vi "Wärmepumpe.VorlauftemperaturSolekreislauf.vi"(0 "Wärmepumpe in":refnum<data-value>, 4 "Rücklauftemperatur Solekreislauf[°C]":dbl, 5 "Error in":errorcluster) -> (14 "Wärmepumpe out":refnum<data-value>, 19 "Error out":errorcluster)   [LabVIEW 2016, in "Wärmepumpe.lvclass"]
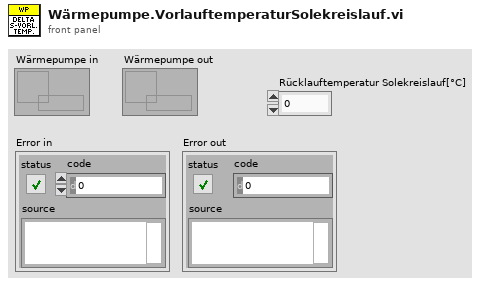
[diagram p1: front panel]
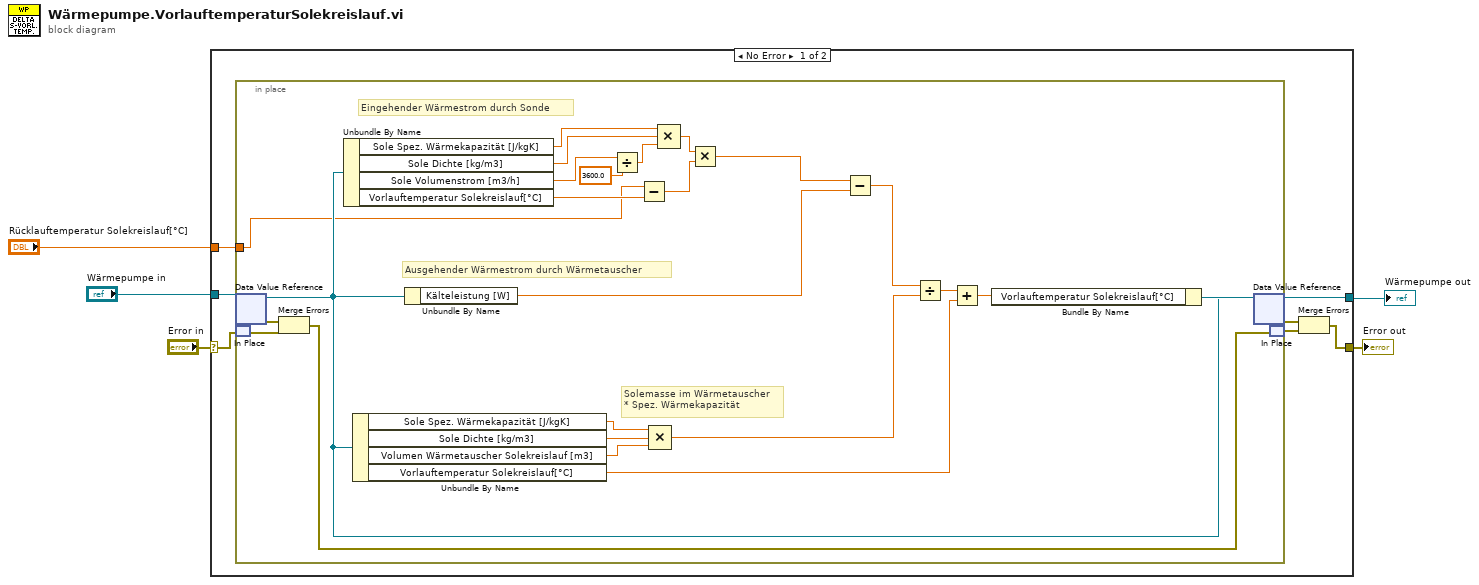
[diagram p0: block diagram]
diagram:
  n1 = case shown="No Error" "Error in" {
    selector: "Error in" -> [w10 w38]
    tunnel: [w9 w37] -> w4
    tunnel: [w8 w38] -> w3
    tunnel: "Wärmepumpe in" -> [w7 w37]
    tunnel: "Rücklauftemperatur Solekreislauf[°C]" -> [w6 _]
    frame No Error {
      n2 = in-place {
        in-place-border: w6 -> [w21]
        # "Solemasse im Wärmetauscher\n* Spez. Wärmekapazität"
        # "Eingehender Wärmestrom durch Sonde"
        # "Ausgehender Wärmestrom durch Wärmetauscher"
        n3 = in-place-dvr #1(w7) -> (w23:refnum<class "Wärmepumpe.lvclass">, w36:errorcluster)
        n4 = in-place-match #2(w10) -> (w35:errorcluster)
        n5 = Merge Errors(w36, w35) -> (w34:errorcluster)
        n6 = Unbundle By Name(w23) -> ("Sole Spez. Wärmekapazität [J/kgK]"=w17:dbl, "Sole Dichte [kg/m3]"=w16:dbl, "Sole Volumenstrom [m3/h]"=w15:dbl, "Vorlauftemperatur Solekreislauf[°C]"=w22:dbl)
        n7 = Unbundle By Name(w23) -> ("Sole Spez. Wärmekapazität [J/kgK]"=w19:dbl, "Sole Dichte [kg/m3]"=w20:dbl, "Volumen Wärmetauscher Solekreislauf [m3]"=w25:dbl, "Vorlauftemperatur Solekreislauf[°C]"=w29:dbl)
        n8 = Unbundle By Name(w23) -> ("Kälteleistung [W]"=w13:dbl)
        n9 = Divide(x=w15, y=3600.0) -> (x/y=w14:dbl)
        n10 = Subtract(x=w21, y=w22) -> (x-y=w26:dbl)
        n11 = Compound Arithmetic op=MULTIPLY(w19, w20, w25) -> (w28:dbl)
        n12 = Compound Arithmetic op=MULTIPLY(w17, w16, w14) -> (w27:dbl)
        n13 = Multiply(x=w27, y=w26) -> (x*y=w24:dbl)
        n14 = Subtract(x=w24, y=w13) -> (x-y=w33:dbl)
        n15 = Divide(x=w33, y=w28) -> (x/y=w32:dbl)
        n16 = Add(x=w32, y=w29) -> (x+y=w31:dbl)
        n17 = Bundle By Name(cluster=w23, "Vorlauftemperatur Solekreislauf[°C]"=w31) -> (w30:refnum<class "Wärmepumpe.lvclass">)
        n18 = in-place-dvr #1(w30) -> (w9:refnum<data-value>, w12:errorcluster)
        n19 = in-place-match #2(w34) -> (w11:errorcluster)
      }
      n20 = Merge Errors(w12, w11) -> (w8:errorcluster)
    }
    frame Error {
    }
  }
  "Wärmepumpe out" <- w4
  "Error out" <- w3
